vi "Digital Pulse Acquire.vi"() -> ()   [LabVIEW 2019, in "Part of Main VIs.lvlib" / "Tachometer Library.lvlib"]
uses:
  ccounter Input Type_TypeDef.ctl
  <vilib>/Utility/error.llb/DialogType.ctl
  692b934c-ada2-4771-a20b-de68b910c917.vi
  <vilib>/DAQmx/read.llb/DAQmx Read (Counter 1D DBL 1Chan NSamp).vi
  de4a30f1-e00b-4980-9bf9-f34e4a687b90.vi
  83f2a1b9-ae44-4189-94f1-149cd1bf5cda.vi
  bb205f37-9733-478c-ac83-00c2c1e1fc19.vi
  <vilib>/DAQmx/read.llb/DAQmx Read (Analog 1D DBL 1Chan NSamp).vi
  <extravilib>/ChannelInstances/Tag-a[.](dbl)/Read With Abort.vi
  <extravilib>/ChannelInstances/Tag-a[.](dbl)/Write With Abort.vi
  <vilib>/DAQmx/create/channels.llb/DAQmx Create Channel (AI-Voltage-Basic).vi
  <vilib>/DAQmx/configure/timing.llb/DAQmx Timing (Sample Clock).vi
  <vilib>/DAQmx/miscellaneous.llb/DAQmx Fill In Error Info.vi
  <extravilib>/ChannelInstances/Tag-a[.](dbl)/Instantiate.vi
  <extravilib>/ChannelInstances/Tag-a[.](dbl)/EndpointRead.vi
  <extravilib>/ChannelInstances/Tag-a[.](dbl)/Endpoint.vi
  <vilib>/DAQmx/create/channels.llb/DAQmx Create Channel (CI-Period).vi
  <vilib>/DAQmx/configure/timing.llb/DAQmx Timing (Implicit).vi
  <vilib>/DAQmx/create/channels.llb/DAQmx Create Channel (CI-Semi Period).vi
  <vilib>/DAQmx/create/channels.llb/DAQmx Create Channel (CI-Frequency).vi
  <vilib>/DAQmx/create/channels.llb/DAQmx Create Channel (CI-Count Edges).vi
  <vilib>/DAQmx/create/channels.llb/DAQmx Create Channel (CI-Pulse Width).vi
  Tachometer Library.lvlib
  <resource>/objmgr/daqmx.rc
  <extravilib>/ChannelInstances/Tag-a[.](dbl).lvlib
panel:
  out "Average":dbl
  out "element":dbl
  out "Pulse per 100ms":dbl[](array[numeric])
  out "RPM":dbl[](array[numeric])
  out "Pulse per sec":dbl[](array[numeric])
  out "data":dbl[](array[numeric]) format="%0.2f"
  in  "Stop":bool
  out "SampClk.Timebase.Src":tag
  out "SampClk.Src":tag
  out "Waveform Graph 2":waveform(dbl)(graph)
  out "Waveform Graph":waveform(dbl)(graph)
  in  "samples per channel":i32=1000
  in  "Counter Physical Channel":tag="PXI-6624/ctr1"
  out "Measurement Chart":dbl[](graph)
  out "SampClk.MaxRate":dbl
  out "Amplitude Chart":dbl[](graph)
  in  "Sample Rate":dbl=5000.0
  in  "Sample Clock Source":tag="OnboardClock"
  in  "Terminal Configuration":i32(ring)=-1 items=["default"=-1, "RSE"=10083, "NRSE"=10078, "Differential"=10106, "Pseudodifferential"=12529]
  in  "Max Voltage":dbl=5.0
  in  "Min Voltage":dbl=-5.0
  in  "Physical Channel":tag="PXIe-4304/ai0"
  out "Actual Sample Rate":dbl=1000.0 format="%0.2f"
  in  "Counter Input Type":T1=enum."Frequency"
  in  "Period Input Terminal":tag="/PXI-6624/PFI34"
  in  "Max Period":dbl=0.1 format="%0.6f"
  in  "Min Period":dbl=1e-06 format="%0.6f"
  in  "Period Input Terminal 2":tag="/PXI-6624/PFI34"
  out "CI.CountEdges.Dir":i32(ring)=10128 items=["Count Up"=10128, "Count Down"=10124, "Externally Controlled"=10326]
  in  "Min Frequency":dbl=2.0 format="%0.6f"
  in  "Max Frequency":dbl=100.0 format="%0.6f"
  out "CI.CtrTimebaseSrc":tag
  in  "Frequency Input Terminal":tag="/PXI-6624/PFI34"
  in  "Pulse Width Input Terminal":tag="/PXI-6624/PFI34"
  in  "Min Pulse Width":dbl=1e-06 format="%0.6f"
  in  "Max Pulse Width":dbl=0.1 format="%0.6f"
  in  "Min Semi-Period":dbl=1e-06 format="%0.6f"
  in  "Max Semi-Period":dbl=0.1 format="%0.6f"
  in  "Semi-Period Input Terminal":tag="/PXI-6624/PFI34"
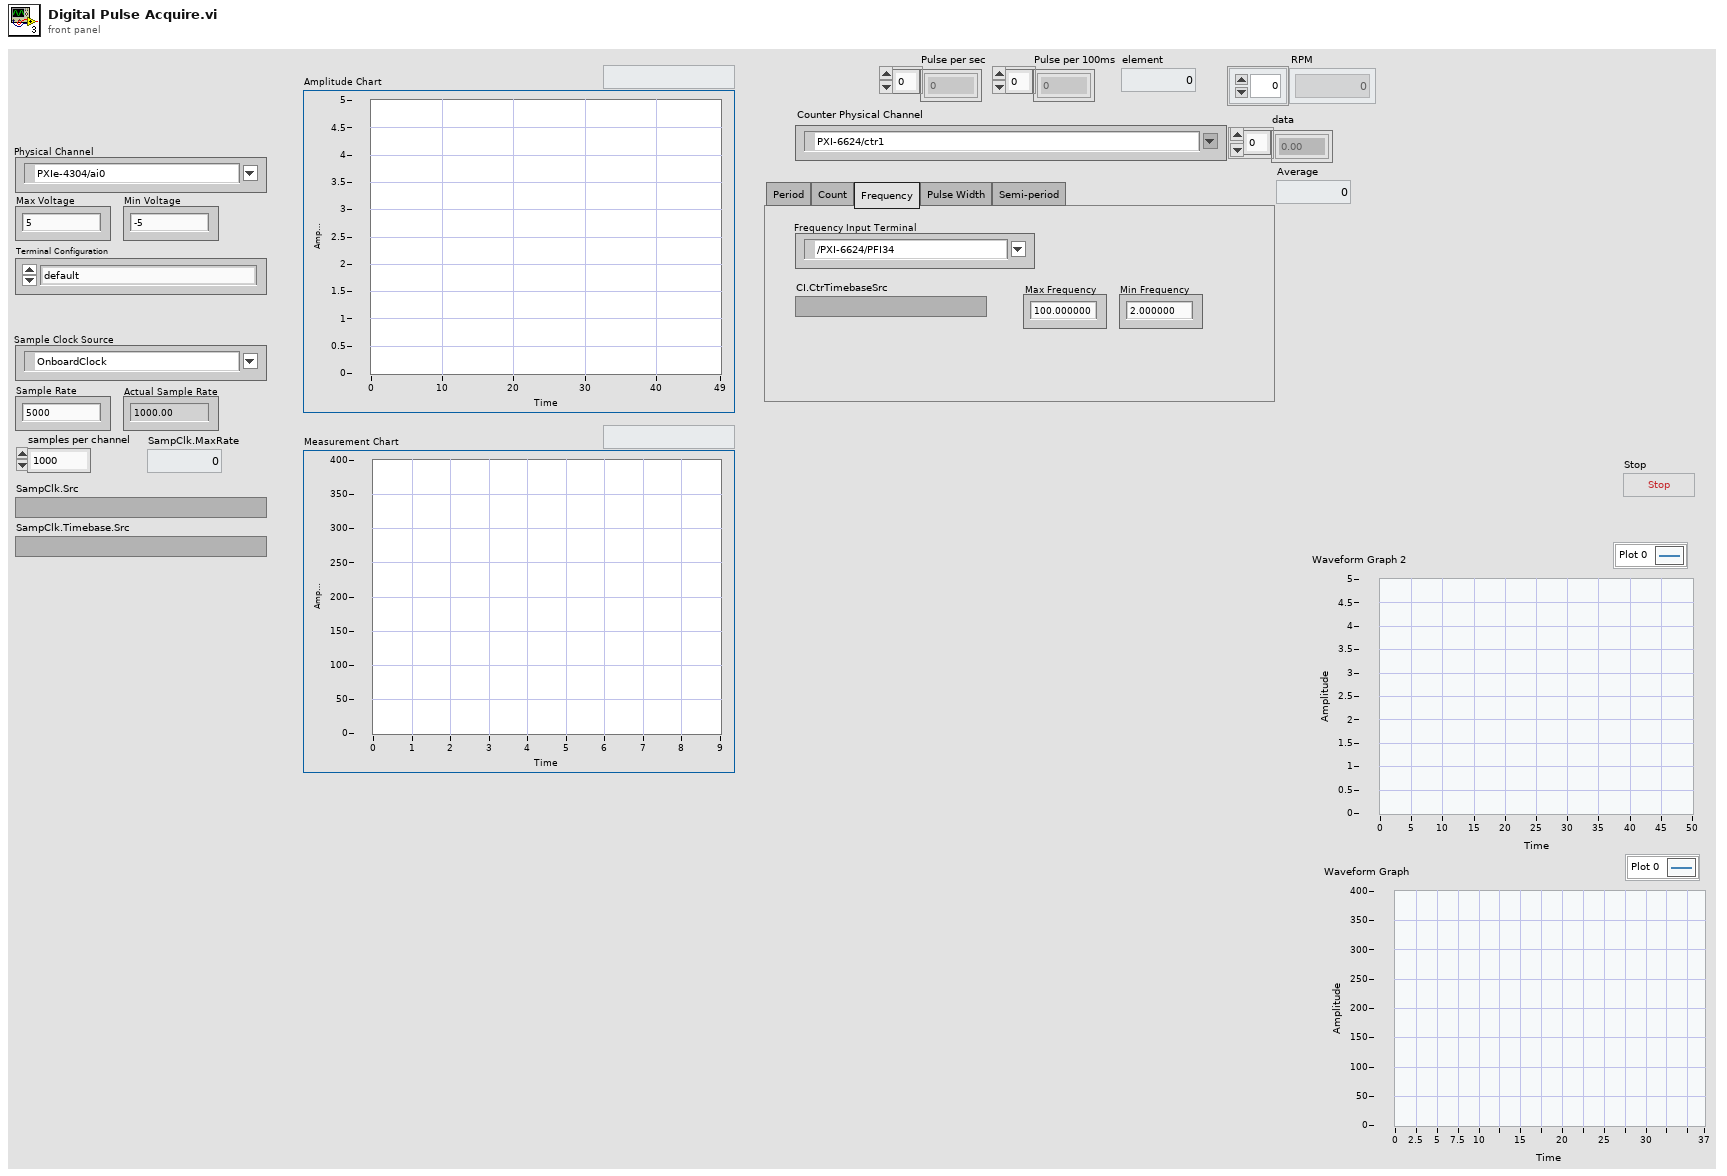
[diagram p1: front panel]
types:
  T1 = typedef "ccounter Input Type_TypeDef.ctl" = enum32{"Period", "Count", "Frequency", "Pulse Width", "Semi-period"}
  T2 = typedef "DialogType.ctl" = u16
  T3 = typedef "Tag-a[.](dbl).lvlib/))Channel.ctl" = refnum<queue>
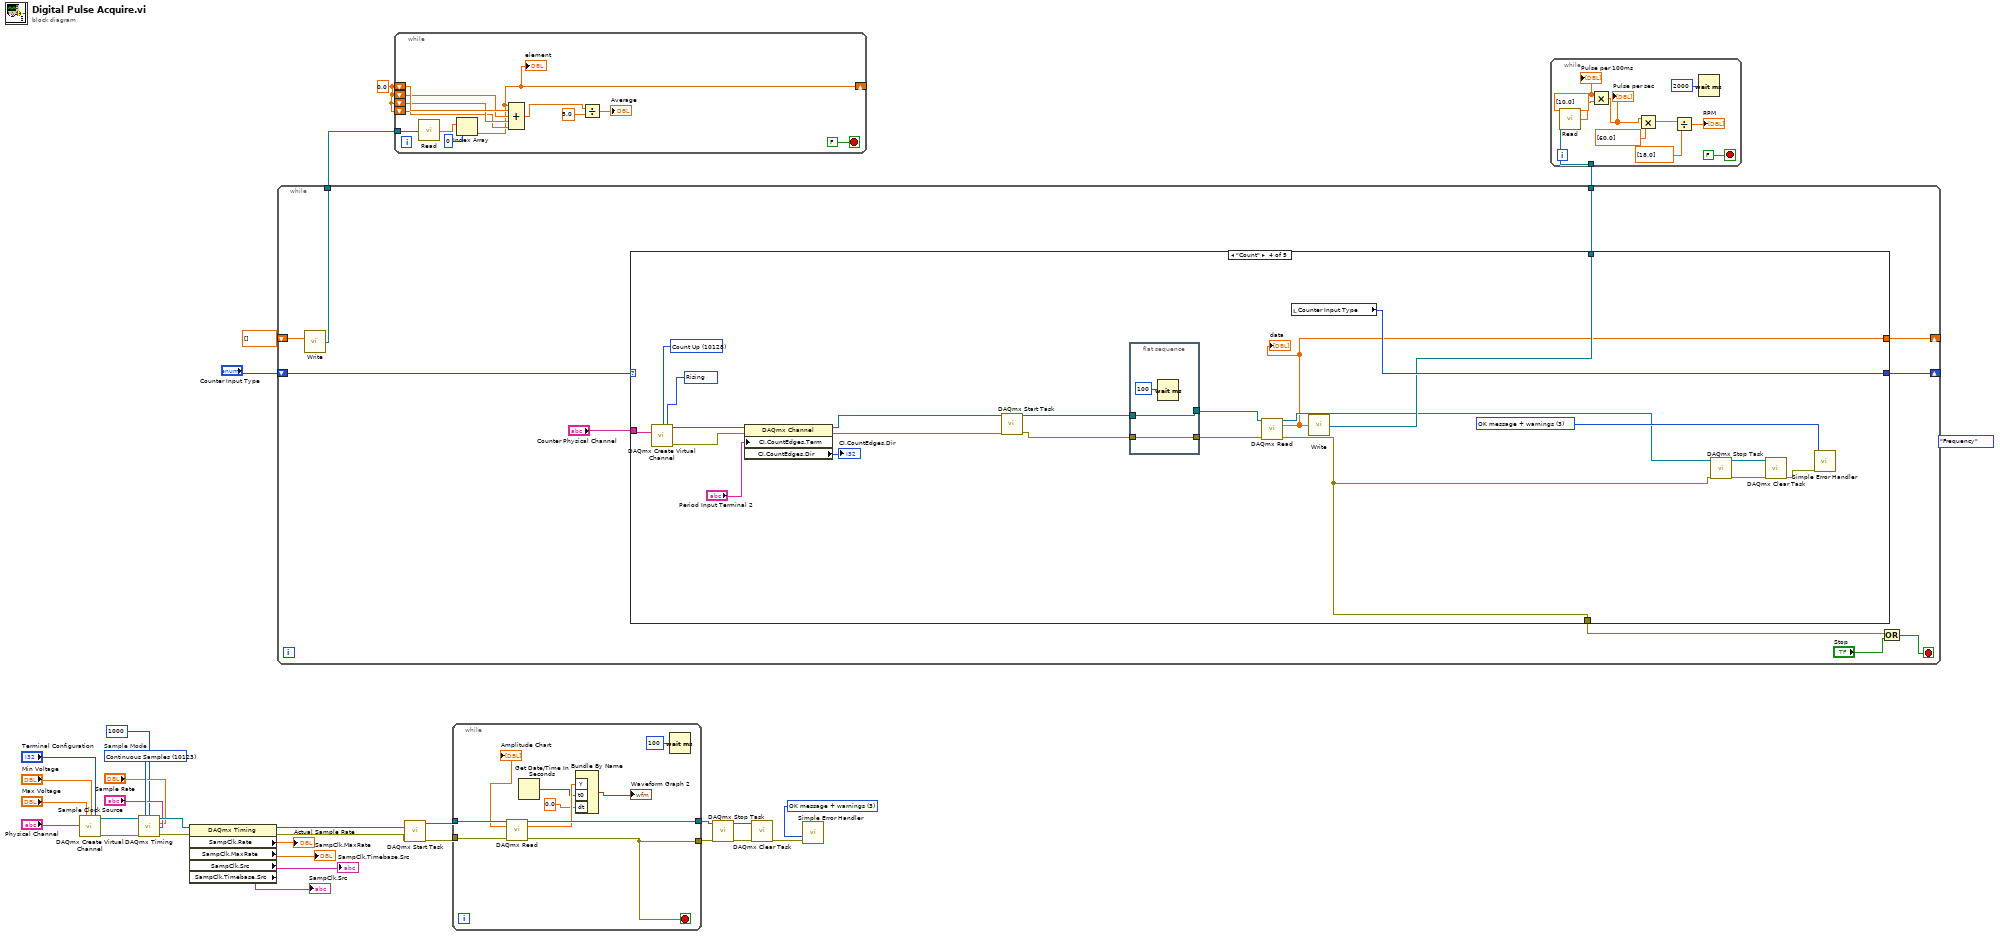
[diagram p0: block diagram]
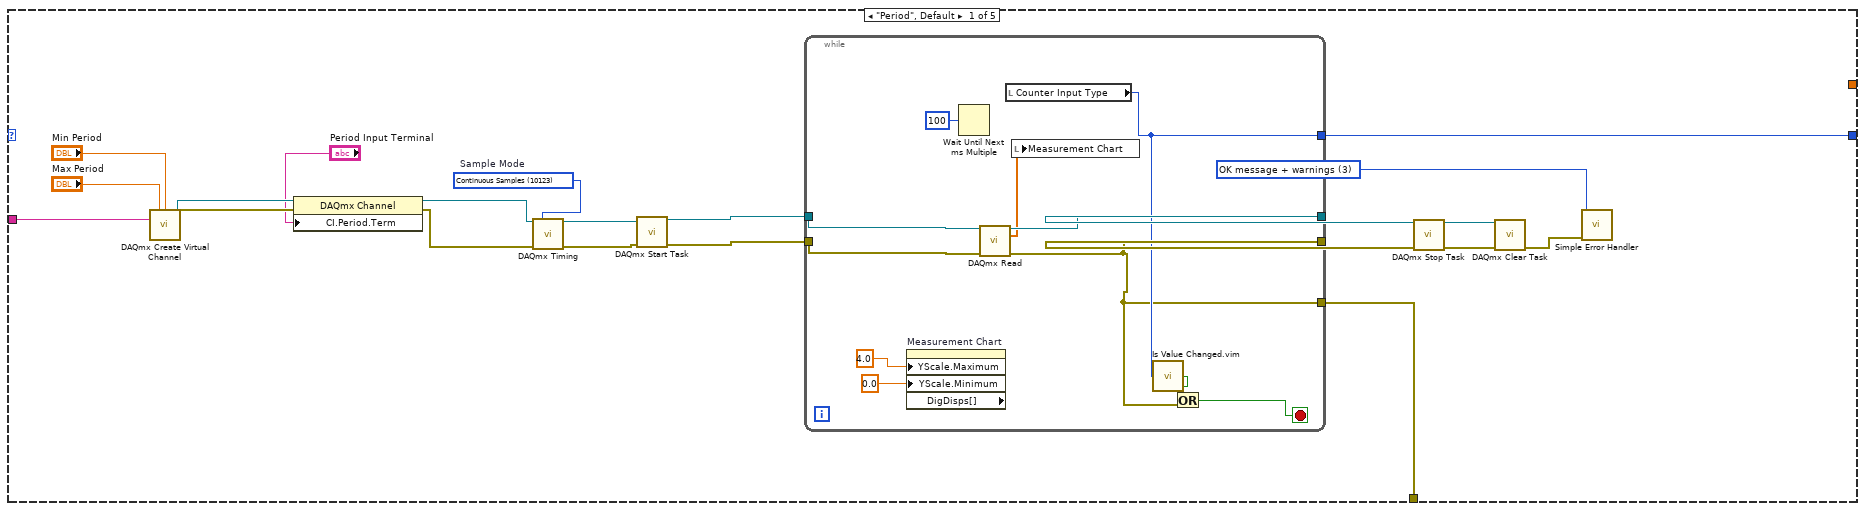
[diagram p2: hidden frame]
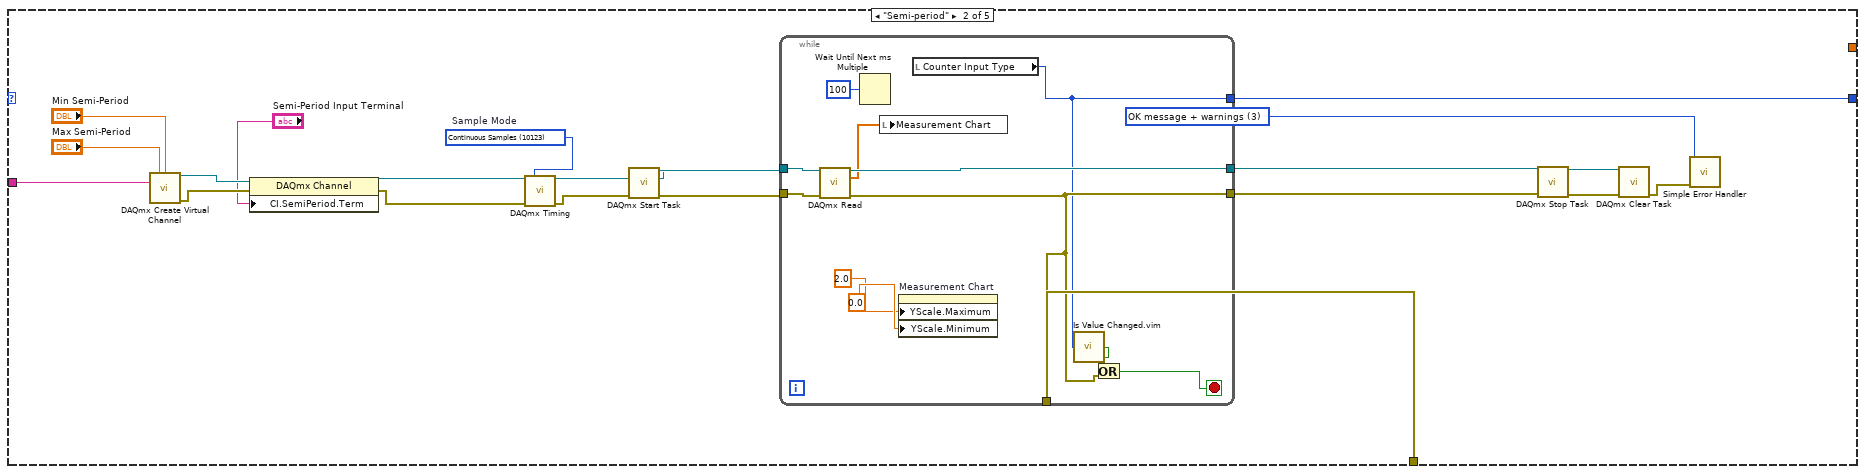
[diagram p3: hidden frame]
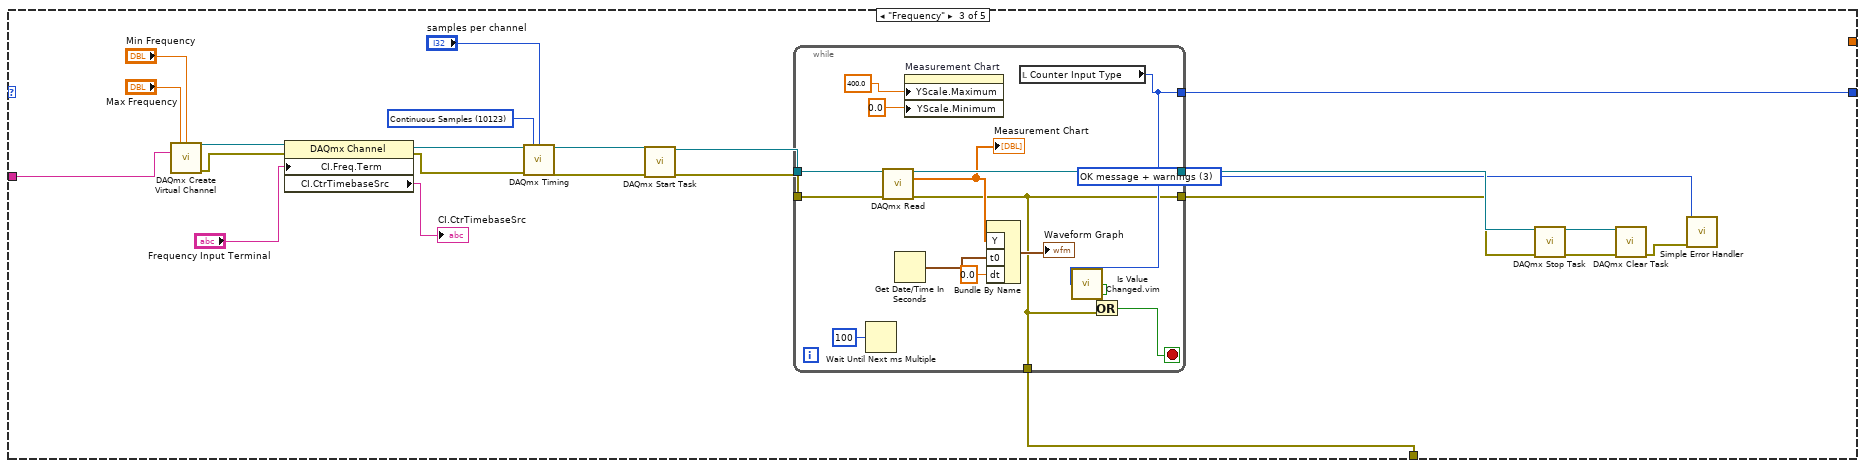
[diagram p4: hidden frame]
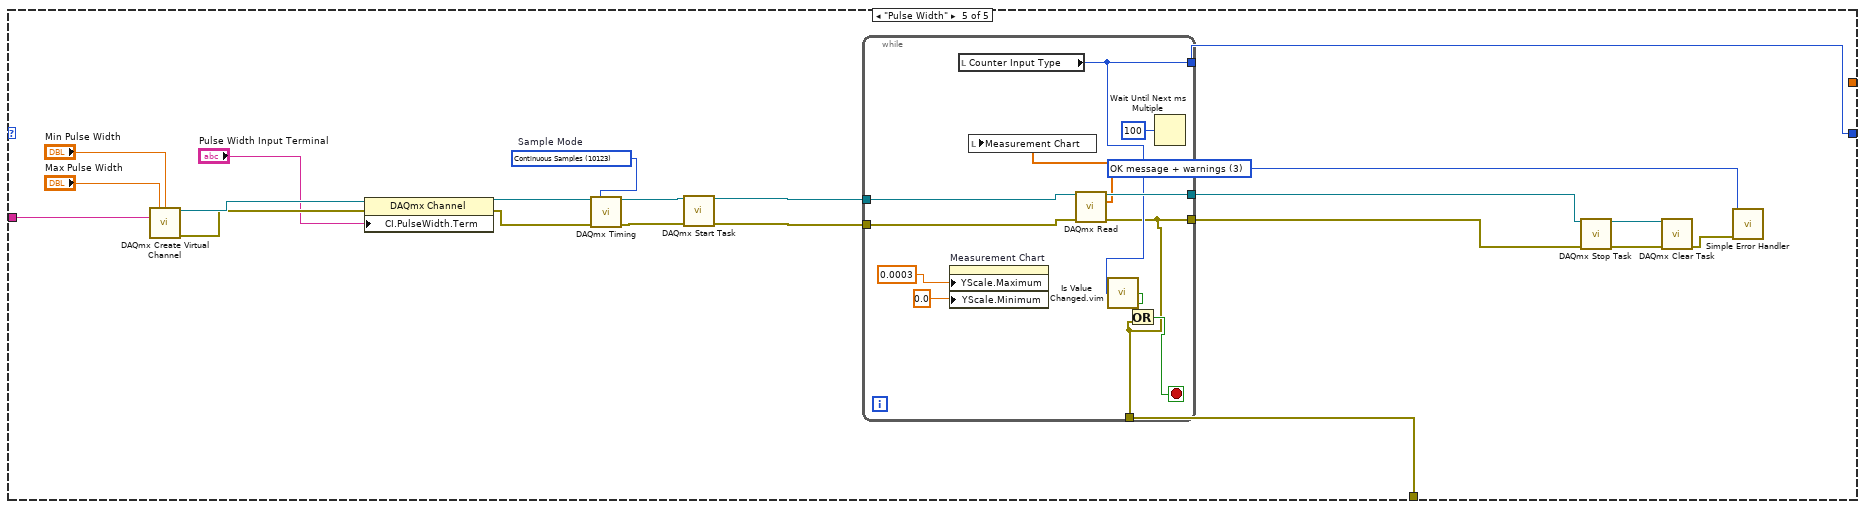
[diagram p5: hidden frame]
diagram:
  w7 = 0.0 ("Waveform")
  (unwired) ccounter_Input_Type_TypeDef."Frequency" ("Counter Input Type")
  w25 = 10123 items=["Finite Samples"=10178, "Continuous Samples"=10123, "Hardware Timed Single Point"=12522]  # Sample Mode
  w31 = T2 3 items=["no dialog", "OK message", "continue or stop message", "OK message + warnings", "continue/stop + warnings"] ("type of dialog (OK msg:1)")
  n1 = call-poly <vilib>:"DAQmx Create Virtual Channel.vi"("maximum value"="Max Voltage", "minimum value"="Min Voltage", "input terminal configuration"="Terminal Configuration", "physical channels"="Physical Channel") -> ("task out"=w23:refnum<k21>, "error out"=w24:errorcluster)  [unwired: 10 in]
  n2 = call-poly <vilib>:"DAQmx Timing.vi"("task/channels in"=w23, "sample mode"=w25, "samples per channel"=1000, "rate"="Sample Rate", "source"="Sample Clock Source", "error in"=w24) -> ("task out"=w27:refnum<k21>, "error out"=w26:errorcluster)  [unwired: 8 in]
  n3 = property class="DAQmx Timing"(reference=w27, error in=w26) -> (reference out=w6:refnum<k21>, error out=w5:errorcluster, "SampClk.Rate"=→"Actual Sample Rate":dbl, "SampClk.MaxRate"=→"SampClk.MaxRate":dbl, "SampClk.Src"=→"SampClk.Src":tag, "SampClk.Timebase.Src"=→"SampClk.Timebase.Src":tag)
  n4 = while {
    shift-right: [w36] -> _
    shift-left: "Counter Input Type" -> [w38]
    tunnel: [w35] -> w10
    shift-right: [w34] -> _
    shift-left: dbl[] [] ("data") -> [w33]
    tunnel: [w32] -> w8
    stop <- w39 stop-if-true
    n5 = call <extravilib>:"Write.vi"("element"=w33) -> ("channel"=w32:T3)  [unwired: 1 out]
    n6 = case shown="\"Count\"" w38 {
      tunnel: [w44 w76 w107 w148 w170] -> w40
      tunnel: "Counter Physical Channel" -> [w43 w75 w109 w159 w169]
      tunnel: [w42 w74 w108 w154 w168] -> w36
      tunnel: [_ _ _ w150 _] -> w35
      tunnel: [_ _ _ w143 _] -> w34
      frame "Period", Default {
        w47 = T2 3 items=["no dialog", "OK message", "continue or stop message", "OK message + warnings", "continue/stop + warnings"] ("type of dialog (OK msg:1)")
        w57 = 10123 items=["Finite Samples"=10178, "Continuous Samples"=10123, "Hardware Timed Single Point"=12522]  # Sample Mode
        n7 = call-poly <vilib>:"DAQmx Create Virtual Channel.vi"("maximum value"="Max Period", "minimum value"="Min Period", "counter"=w43) -> ("task out"=w62:refnum<k21>, "error out"=w61:errorcluster)  [unwired: 11 in]
        n8 = property class="DAQmx Channel"(reference=w62, error in=w61, "CI.Period.Term"="Period Input Terminal") -> (reference out=w56:refnum<k21>, error out=w55:errorcluster)
        n9 = call-poly <vilib>:"DAQmx Timing.vi"("task/channels in"=w56, "sample mode"=w57, "error in"=w55) -> ("task out"=w52:refnum<k21>, "error out"=w51:errorcluster)  [unwired: 11 in]
        n10 = call <vilib>:"DAQmx Start Task.vi"("task/channels in"=w52, "error in"=w51) -> ("task out"=w53:refnum<k21>, "error out"=w54:errorcluster)  [unwired: 12 in]
        n11 = while {
          tunnel: w54 -> [w73]
          tunnel: [w64] -> w45
          tunnel: w53 -> [w72]
          tunnel: [w71] -> w46
          tunnel: [w64] -> w44
          tunnel: [w65] -> w42
          stop <- w63 stop-if-true
          n12 = property on="Measurement Chart" class="WFChart (strict)" props=["YScale", "Maximum", "YScale", "Minimum", "DigDisps[]"]("YScale.Maximum"=4.0 ("Y Scale.Range:Maximum"), "YScale.Minimum"=0.0 ("Y Scale.Range:Minimum")) -> ()  [unwired: 2 in, 3 out]
          n13 = Wait Until Next ms Multiple(millisecond multiple=u32 100) -> ()  [unwired: 1 out]
          n14 = call-poly <vilib>:"DAQmx Read.vi"("task/channels in"=w72, "error in"=w73) -> ("task out"=w71:refnum<k21>, "data"=w69:dbl[], "error out"=w64:errorcluster)  [unwired: 11 in]
          n15 = local read "Counter Input Type"() -> (w65:T1)
          n16 = local write "Measurement Chart"(w69) -> ()
          n17 = call "Is Value Changed.vim"("value"=w65) -> ("changed or first call?"=w66:bool)
          n18 = Or(x=w66, y=w64) -> (x .or. y?=w63:bool)
        }
        n19 = call <vilib>:"DAQmx Stop Task.vi"("task/channels in"=w46, "error in"=w45) -> ("task out"=w50:refnum<k21>, "error out"=w49:errorcluster)  [unwired: 12 in]
        n20 = call <vilib>:"DAQmx Clear Task.vi"("task in"=w50, "error in"=w49) -> ("error out"=w48:errorcluster)  [unwired: 13 in]
        n21 = call <vilib>:"Simple Error Handler.vi"("type of dialog (OK msg:1)"=w47, "error in (no error)"=w48) -> ()  [unwired: 3 in, 5 out]
      }
      frame "Semi-period" {
        w79 = T2 3 items=["no dialog", "OK message", "continue or stop message", "OK message + warnings", "continue/stop + warnings"] ("type of dialog (OK msg:1)")
        w89 = 10123 items=["Finite Samples"=10178, "Continuous Samples"=10123, "Hardware Timed Single Point"=12522]  # Sample Mode
        n22 = call-poly <vilib>:"DAQmx Create Virtual Channel.vi"("maximum value"="Max Semi-Period", "minimum value"="Min Semi-Period", "counter"=w75) -> ("task out"=w94:refnum<k21>, "error out"=w93:errorcluster)  [unwired: 11 in]
        n23 = property class="DAQmx Channel"(reference=w94, error in=w93, "CI.SemiPeriod.Term"="Semi-Period Input Terminal") -> (reference out=w88:refnum<k21>, error out=w87:errorcluster)
        n24 = call-poly <vilib>:"DAQmx Timing.vi"("task/channels in"=w88, "sample mode"=w89, "error in"=w87) -> ("task out"=w84:refnum<k21>, "error out"=w83:errorcluster)  [unwired: 11 in]
        n25 = call <vilib>:"DAQmx Start Task.vi"("task/channels in"=w84, "error in"=w83) -> ("task out"=w85:refnum<k21>, "error out"=w86:errorcluster)  [unwired: 12 in]
        n26 = while {
          tunnel: w86 -> [w105]
          tunnel: [w96] -> w77
          tunnel: w85 -> [w104]
          tunnel: [w103] -> w78
          tunnel: [w96] -> w76
          tunnel: [w95] -> w74
          stop <- w97 stop-if-true
          n27 = call-poly <vilib>:"DAQmx Read.vi"("task/channels in"=w104, "error in"=w105) -> ("task out"=w103:refnum<k21>, "data"=w102:dbl[], "error out"=w96:errorcluster)  [unwired: 11 in]
          n28 = Wait Until Next ms Multiple(millisecond multiple=u32 100) -> ()  [unwired: 1 out]
          n29 = local write "Measurement Chart"(w102) -> ()
          n30 = property on="Measurement Chart" class="WFChart (strict)"("YScale.Maximum"=2.0 ("Y Scale.Range:Maximum"), "YScale.Minimum"=0.0 ("Y Scale.Range:Minimum")) -> ()  [unwired: 2 in, 2 out]
          n31 = local read "Counter Input Type"() -> (w95:T1)
          n32 = call "Is Value Changed.vim"("value"=w95) -> ("changed or first call?"=w98:bool)
          n33 = Or(x=w98, y=w96) -> (x .or. y?=w97:bool)
        }
        n34 = call <vilib>:"DAQmx Stop Task.vi"("task/channels in"=w78, "error in"=w77) -> ("task out"=w82:refnum<k21>, "error out"=w81:errorcluster)  [unwired: 12 in]
        n35 = call <vilib>:"DAQmx Clear Task.vi"("task in"=w82, "error in"=w81) -> ("error out"=w80:errorcluster)  [unwired: 13 in]
        n36 = call <vilib>:"Simple Error Handler.vi"("type of dialog (OK msg:1)"=w79, "error in (no error)"=w80) -> ()  [unwired: 3 in, 5 out]
      }
      frame "Frequency" {
        w112 = 10123 items=["Finite Samples"=10178, "Continuous Samples"=10123, "Hardware Timed Single Point"=12522] ("sample mode")
        w113 = T2 3 items=["no dialog", "OK message", "continue or stop message", "OK message + warnings", "continue/stop + warnings"] ("type of dialog (OK msg:1)")
        n37 = call-poly <vilib>:"DAQmx Create Virtual Channel.vi"("maximum value"="Max Frequency", "minimum value"="Min Frequency", "counter"=w109) -> ("task out"=w126:refnum<k21>, "error out"=w125:errorcluster)  [unwired: 11 in]
        n38 = property class="DAQmx Channel"(reference=w126, error in=w125, "CI.Freq.Term"="Frequency Input Terminal") -> (reference out=w124:refnum<k21>, error out=w123:errorcluster, "CI.CtrTimebaseSrc"=→"CI.CtrTimebaseSrc":tag)
        n39 = call-poly <vilib>:"DAQmx Timing.vi"("task/channels in"=w124, "sample mode"=w112, "samples per channel"="samples per channel", "error in"=w123) -> ("task out"=w122:refnum<k21>, "error out"=w121:errorcluster)  [unwired: 10 in]
        n40 = call <vilib>:"DAQmx Start Task.vi"("task/channels in"=w122, "error in"=w121) -> ("task out"=w120:refnum<k21>, "error out"=w119:errorcluster)  [unwired: 12 in]
        n41 = while {
          tunnel: w120 -> [w142]
          tunnel: [w140] -> w118
          tunnel: w119 -> [w141]
          tunnel: [w131] -> w117
          tunnel: [w132] -> w108
          tunnel: [w131] -> w107
          stop <- w134 stop-if-true
          n42 = Wait Until Next ms Multiple(millisecond multiple=u32 100) -> ()  [unwired: 1 out]
          n43 = call-poly <vilib>:"DAQmx Read.vi"("task/channels in"=w142, "error in"=w141) -> ("task out"=w140:refnum<k21>, "data"=w135:dbl[], "error out"=w131:errorcluster)  [unwired: 11 in]
          "Measurement Chart" <- w135
          n44 = Get Date/Time In Seconds() -> (seconds since 1Jan1904=w137:timestamp)
          n45 = property on="Measurement Chart" class="WFChart (strict)"("YScale.Maximum"=400.0 ("Y Scale.Range:Maximum"), "YScale.Minimum"=0.0 ("Y Scale.Range:Minimum")) -> ()  [unwired: 2 in, 2 out]
          n46 = Bundle By Name("Y"=w135, "t0"=w137, "dt"=0.0) -> (→"Waveform Graph":waveform(dbl))  [unwired: 1 in]
          n47 = local read "Counter Input Type"() -> (w132:T1)
          n48 = call "Is Value Changed.vim"("value"=w132) -> ("changed or first call?"=w133:bool)
          n49 = Or(x=w133, y=w131) -> (x .or. y?=w134:bool)
        }
        n50 = call <vilib>:"DAQmx Stop Task.vi"("task/channels in"=w118, "error in"=w117) -> ("task out"=w116:refnum<k21>, "error out"=w115:errorcluster)  [unwired: 12 in]
        n51 = call <vilib>:"DAQmx Clear Task.vi"("task in"=w116, "error in"=w115) -> ("error out"=w114:errorcluster)  [unwired: 13 in]
        n52 = call <vilib>:"Simple Error Handler.vi"("type of dialog (OK msg:1)"=w113, "error in (no error)"=w114) -> ()  [unwired: 3 in, 5 out]
      }
      frame "Count" {
        w155 = T2 3 items=["no dialog", "OK message", "continue or stop message", "OK message + warnings", "continue/stop + warnings"] ("type of dialog (OK msg:1)")
        w163 = 10280 items=["Rising"=10280, "Falling"=10171] ("edge")
        w164 = 10128 items=["Count Up"=10128, "Count Down"=10124, "Externally Controlled"=10326] ("count direction")
        n53 = call-poly <vilib>:"DAQmx Create Virtual Channel.vi"("count direction"=w164, "edge"=w163, "counter"=w159) -> ("task out"=w161:refnum<k21>, "error out"=w162:errorcluster)  [unwired: 11 in]
        n54 = property class="DAQmx Channel"(reference=w161, error in=w162, "CI.CountEdges.Term"="Period Input Terminal 2") -> (reference out=w152:refnum<k21>, error out=w151:errorcluster, "CI.CountEdges.Dir"=→"CI.CountEdges.Dir":i32)
        n55 = call <vilib>:"DAQmx Start Task.vi"("task/channels in"=w152, "error in"=w151) -> ("task out"=w146:refnum<k21>, "error out"=w145:errorcluster)  [unwired: 12 in]
        n56 = flat-sequence {
          tunnel: [w166] -> w147
          tunnel: w146 -> [w166]
          tunnel: w145 -> [w165]
          tunnel: [w165] -> w144
          frame #0 {
            n57 = Wait (ms)(milliseconds to wait=u32 100 ("millisecond multiple")) -> ()  [unwired: 1 out]
          }
        }
        n58 = call-poly <vilib>:"DAQmx Read.vi"("task/channels in"=w147, "error in"=w144) -> ("task out"=w149:refnum<k21>, "data"=w143:dbl[], "error out"=w148:errorcluster)  [unwired: 11 in]
        "data" <- w143
        n59 = local read "Counter Input Type"() -> (w154:T1)
        n60 = call <extravilib>:"Write.vi"("element"=w143) -> ("channel"=w150:T3)  [unwired: 1 out]
        n61 = call <vilib>:"DAQmx Stop Task.vi"("task/channels in"=w149, "error in"=w148) -> ("task out"=w158:refnum<k21>, "error out"=w157:errorcluster)  [unwired: 12 in]
        n62 = call <vilib>:"DAQmx Clear Task.vi"("task in"=w158, "error in"=w157) -> ("error out"=w156:errorcluster)  [unwired: 13 in]
        n63 = call <vilib>:"Simple Error Handler.vi"("type of dialog (OK msg:1)"=w155, "error in (no error)"=w156) -> ()  [unwired: 3 in, 5 out]
      }
      frame "Pulse Width" {
        w173 = T2 3 items=["no dialog", "OK message", "continue or stop message", "OK message + warnings", "continue/stop + warnings"] ("type of dialog (OK msg:1)")
        w181 = 10123 items=["Finite Samples"=10178, "Continuous Samples"=10123, "Hardware Timed Single Point"=12522]  # Sample Mode
        n64 = call-poly <vilib>:"DAQmx Create Virtual Channel.vi"("maximum value"="Max Pulse Width", "minimum value"="Min Pulse Width", "counter"=w169) -> ("task out"=w188:refnum<k21>, "error out"=w187:errorcluster)  [unwired: 11 in]
        n65 = property class="DAQmx Channel"(reference=w188, error in=w187, "CI.PulseWidth.Term"="Pulse Width Input Terminal") -> (reference out=w183:refnum<k21>, error out=w182:errorcluster)
        n66 = call-poly <vilib>:"DAQmx Timing.vi"("task/channels in"=w183, "sample mode"=w181, "error in"=w182) -> ("task out"=w178:refnum<k21>, "error out"=w177:errorcluster)  [unwired: 11 in]
        n67 = call <vilib>:"DAQmx Start Task.vi"("task/channels in"=w178, "error in"=w177) -> ("task out"=w180:refnum<k21>, "error out"=w179:errorcluster)  [unwired: 12 in]
        n68 = while {
          tunnel: w179 -> [w198]
          tunnel: [w189] -> w171
          tunnel: w180 -> [w199]
          tunnel: [w197] -> w172
          tunnel: [w189] -> w170
          tunnel: [w191] -> w168
          stop <- w190 stop-if-true
          n69 = property on="Measurement Chart" class="WFChart (strict)"("YScale.Maximum"=0.0003 ("Y Scale.Range:Maximum"), "YScale.Minimum"=0.0 ("Y Scale.Range:Minimum")) -> ()  [unwired: 2 in, 2 out]
          n70 = local read "Counter Input Type"() -> (w191:T1)
          n71 = call-poly <vilib>:"DAQmx Read.vi"("task/channels in"=w199, "error in"=w198) -> ("task out"=w197:refnum<k21>, "data"=w195:dbl[], "error out"=w189:errorcluster)  [unwired: 11 in]
          n72 = local write "Measurement Chart"(w195) -> ()
          n73 = call "Is Value Changed.vim"("value"=w191) -> ("changed or first call?"=w192:bool)
          n74 = Or(x=w192, y=w189) -> (x .or. y?=w190:bool)
          n75 = Wait Until Next ms Multiple(millisecond multiple=u32 100) -> ()  [unwired: 1 out]
        }
        n76 = call <vilib>:"DAQmx Stop Task.vi"("task/channels in"=w172, "error in"=w171) -> ("task out"=w176:refnum<k21>, "error out"=w175:errorcluster)  [unwired: 12 in]
        n77 = call <vilib>:"DAQmx Clear Task.vi"("task in"=w176, "error in"=w175) -> ("error out"=w174:errorcluster)  [unwired: 13 in]
        n78 = call <vilib>:"Simple Error Handler.vi"("type of dialog (OK msg:1)"=w173, "error in (no error)"=w174) -> ()  [unwired: 3 in, 5 out]
      }
    }
    n79 = Or(x=w40, y="Stop") -> (x .or. y?=w39:bool)
  }
  n80 = while {
    tunnel: w8 -> [w211]
    shift-right: [w200] -> _
    shift-left: w7 -> [w208]
    shift-left: w7 -> [w207]
    shift-left: w7 -> [w206]
    shift-left: w7 -> [w205]
    stop <- FALSE stop-if-true
    n81 = call <extravilib>:"Read.vi"("channel"=w211) -> ("element"=w209:dbl[])  [unwired: 1 in, 1 out]
    n82 = Index Array(array=w209, index=0) -> (element=w200:dbl)
    "element" <- w200
    n83 = Compound Arithmetic op=ADD(w200, w208, w207, w206, w205) -> (w203:dbl)
    n84 = Divide(x=w203, y=5.0) -> (x/y=→"Average":dbl)
  }
  n85 = call <vilib>:"DAQmx Start Task.vi"("task/channels in"=w6, "error in"=w5) -> ("task out"=w2:refnum<k21>, "error out"=w1:errorcluster)  [unwired: 12 in]
  n86 = while {
    tunnel: w1 -> [w218]
    tunnel: [w212] -> w3
    tunnel: w2 -> [w219]
    tunnel: [w220] -> w4
    stop <- w212 stop-if-true
    n87 = call-poly <vilib>:"DAQmx Read.vi"("task/channels in"=w219, "error in"=w218) -> ("task out"=w220:refnum<k21>, "data"=w216:dbl[], "error out"=w212:errorcluster)  [unwired: 11 in]
    "Amplitude Chart" <- w216
    n88 = Get Date/Time In Seconds() -> (seconds since 1Jan1904=w215:timestamp)
    n89 = Bundle By Name("Y"=w216, "t0"=w215, "dt"=0.0) -> (→"Waveform Graph 2":waveform(dbl))  [unwired: 1 in]
    n90 = Wait (ms)(milliseconds to wait=u32 100) -> ()  [unwired: 1 out]
  }
  n91 = call <vilib>:"DAQmx Stop Task.vi"("task/channels in"=w4, "error in"=w3) -> ("task out"=w30:refnum<k21>, "error out"=w29:errorcluster)  [unwired: 12 in]
  n92 = call <vilib>:"DAQmx Clear Task.vi"("task in"=w30, "error in"=w29) -> ("error out"=w28:errorcluster)  [unwired: 13 in]
  n93 = call <vilib>:"Simple Error Handler.vi"("type of dialog (OK msg:1)"=w31, "error in (no error)"=w28) -> ()  [unwired: 3 in, 5 out]
  n94 = while {
    tunnel: w10 -> [w230]
    stop <- FALSE stop-if-true
    n95 = call <extravilib>:"Read.vi"("channel"=w230) -> ("element"=w222:dbl[])  [unwired: 1 in, 1 out]
    "Pulse per 100ms" <- w222
    n96 = Multiply(x=w222, y=dbl[] [10.0]) -> (x*y=w223:dbl[])
    "Pulse per sec" <- w223
    n97 = Multiply(x=w223, y=dbl[] [60.0]) -> (x*y=w227:dbl[])
    n98 = Divide(x=w227, y=dbl[] [18.0]) -> (x/y=→"RPM":dbl[])
    n99 = Wait (ms)(milliseconds to wait=u32 2000) -> ()  [unwired: 1 out]
  }
